vi "binary sub.vi"(8 "Tens?":bool, 9 "order":u8, 10 "Time Stamp":timestamp, 11 "time format string (%c)":string) -> (2 "Time Stamp 2":timestamp, 3 "Array":bool[](array[boolean]))   [LabVIEW 2014]
uses:
  <vilib>/myRIO/Instrument Drivers/Onboard IO/DIO/typedefs/DIO Reference.ctl
  <vilib>/myRIO/Common/Instrument Driver Framework/Utilities/typedefs/myRIO Generic Hardware Reference.ctl
  <vilib>/myRIO/Common/Instrument Driver Framework/Utilities/typedefs/Hardware Version Enum.ctl
  <vilib>/myRIO/Common/Instrument Driver Framework/Utilities/typedefs/myRIO v1.0 Reference.ctl
  <vilib>/myRIO/Common/Instrument Driver Framework/Utilities/typedefs/Generic FPGA Reference.ctl
  <vilib>/myRIO/Common/Instrument Driver Framework/myRIO v1.0/DIO/typedefs/DIO Channels List.ctl
  <vilib>/myRIO/Common/Instrument Driver Framework/myRIO v1.0/DIO/typedefs/DIO Channels Enum.ctl
  <vilib>/userdefined/High Color/nirio_resource_hc.ctl
  <vilib>/myRIO/Common/Instrument Driver Framework/Utilities/vis/Is FPGA Ref Available.vi
  <vilib>/myRIO/Common/Instrument Driver Framework/myRIO v1.0/DIO/vis/myRIO v1.1 Open DIO.vi
  <vilib>/myRIO/Instrument Drivers/Onboard IO/DIO/vis/Write.vi
  <vilib>/myRIO/Common/Instrument Driver Framework/Utilities/vis/Validate Channels.vi
  <vilib>/myRIO/Common/Instrument Driver Framework/myRIO v1.0/DIO/vis/myRIO v1.0 Reserve DIO.vi
  <vilib>/myRIO/Common/Instrument Driver Framework/myRIO v1.0/Resource Manager/vis/myRIO v1.0 Reserve Channel List.vi
  <vilib>/myRIO/Common/Instrument Driver Framework/myRIO v1.0/DIO/vis/myRIO v1.0 Build MUX Configuration DIO.vi
  <vilib>/myRIO/Common/Instrument Driver Framework/myRIO v1.0/Resource Manager/vis/myRIO v1.0 Reserve Channel.vi
  <vilib>/myRIO/Common/Instrument Driver Framework/myRIO v1.0/Resource Manager/vis/myRIO v1.0 Unreserve Channel.vi
  <vilib>/myRIO/Common/Instrument Driver Framework/myRIO v1.0/Resource Manager/vis/myRIO v1.0 Create Configuration List.vi
  <vilib>/myRIO/Common/Instrument Driver Framework/myRIO v1.0/Resource Manager/vis/myRIO v1.0 Build Mutex Name.vi
  <vilib>/Utility/VariantDataType/GetNumericInfo.vi
  <vilib>/Utility/error.llb/Error Cluster From Error Code.vi
  <vilib>/myRIO/Common/Instrument Driver Framework/myRIO v1.0/myRIO v1.1 Open.vi
  <vilib>/myRIO/Common/Instrument Driver Framework/Utilities/vis/IO Manager.vi
  <vilib>/myRIO/Common/Instrument Driver Framework/Utilities/vis/Configuration Manager.vi
  <vilib>/myRIO/Common/Instrument Driver Framework/myRIO v1.0/Resource Manager/vis/myRIO v1.0 Configure IO.vi
  <vilib>/myRIO/Common/Instrument Driver Framework/myRIO v1.0/myRIO v1.0 Close.vi
  <vilib>/myRIO/Common/Instrument Driver Framework/myRIO v1.0/DIO/vis/myRIO v1.0 Write DIO.vi
  <vilib>/myRIO/Express VI/Onboard IO/DO/DO Express VI.xnode
  <vilib>/myRIO/Instrument Drivers/Onboard IO/DIO/vis/myRIO DIO Open.xnode
  <vilib>/myRIO/Instrument Drivers/Onboard IO/DIO/DIO.lvlib
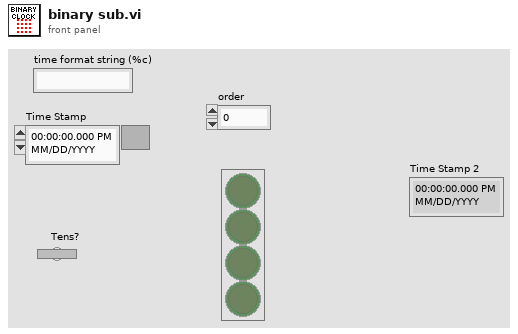
[diagram p1: front panel]
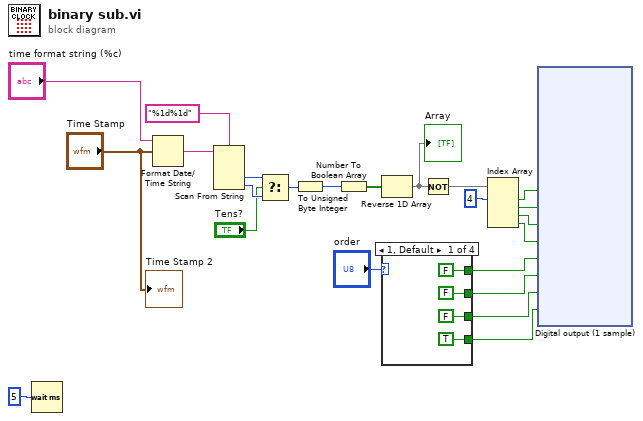
[diagram p0: block diagram]
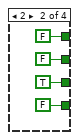
[diagram p2: hidden frame]
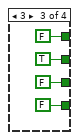
[diagram p3: hidden frame]
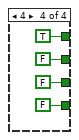
[diagram p4: hidden frame]
diagram:
  n1 = Wait (ms)(milliseconds to wait=u32 5) -> ()  [unwired: 1 out]
  n2 = Format Date/Time String(time format string (%c)="time format string (%c)", seconds (now)="Time Stamp") -> (date/time string=w22:string)  [unwired: 1 in]
  n3 = Scan From String(format string="%1d%1d", input string=w22) -> (output 1=w8:i32, output 2=w7:i32)  [unwired: 4 in, 3 out]
  n4 = Select(t=w8, s="Tens?", f=w7) -> (s? t:f=w9:i32)
  n5 = To Unsigned Byte Integer(number=w9) -> (unsigned 8bit integer=w21:u8)
  n6 = Number To Boolean Array(number=w21) -> (Boolean array=w15:bool[])
  n7 = Reverse 1D Array(array=w15) -> (reversed array=w13:bool[])
  "Array" <- w13
  n8 = case shown="1, Default" "order" {
    tunnel: [FALSE FALSE FALSE TRUE] -> w4
    tunnel: [FALSE FALSE TRUE FALSE] -> w3
    tunnel: [FALSE TRUE FALSE FALSE] -> w2
    tunnel: [TRUE FALSE FALSE FALSE] -> w1
    frame 1, Default {
    }
    frame 2 {
    }
    frame 3 {
    }
    frame 4 {
    }
  }
  n9 = Not(x=w13) -> (.not. x?=w14:bool[])
  n10 = Index Array(array=w14, index #1=4 ("index")) -> (element #1=w19:bool, element #2=w18:bool, element #3=w17:bool, element #4=w16:bool)  [unwired: 3 in]
  n11 = xnode "Digital output (1 sample)"("B/DIO0 (Pin 11)"=w19, "B/DIO1 (Pin 13)"=w18, "B/DIO2 (Pin 15)"=w17, "B/DIO3 (Pin 17)"=w16, "B/DIO4 (Pin 19)"=w4, "B/DIO5 (Pin 21)"=w3, "B/DIO6 (Pin 23)"=w2, "B/DIO7 (Pin 25)"=w1) -> ()  [unwired: 1 in, 1 out]
  "Time Stamp 2" <- "Time Stamp"
